vi "odczyt listy zdjec.vi"(5 "error in (no error)":errorcluster) -> (0 "error out":errorcluster, 1 "Nr zdjecia":i32[](array[numeric]), 2 "fps":i32[](array[numeric]), 3 "lista zdjec":string[](array[string]), 4 "sciezka do zdjec":path caption="selected path", 6 "godzina ze zdjecia":string[](array[string]))   [LabVIEW 2009]
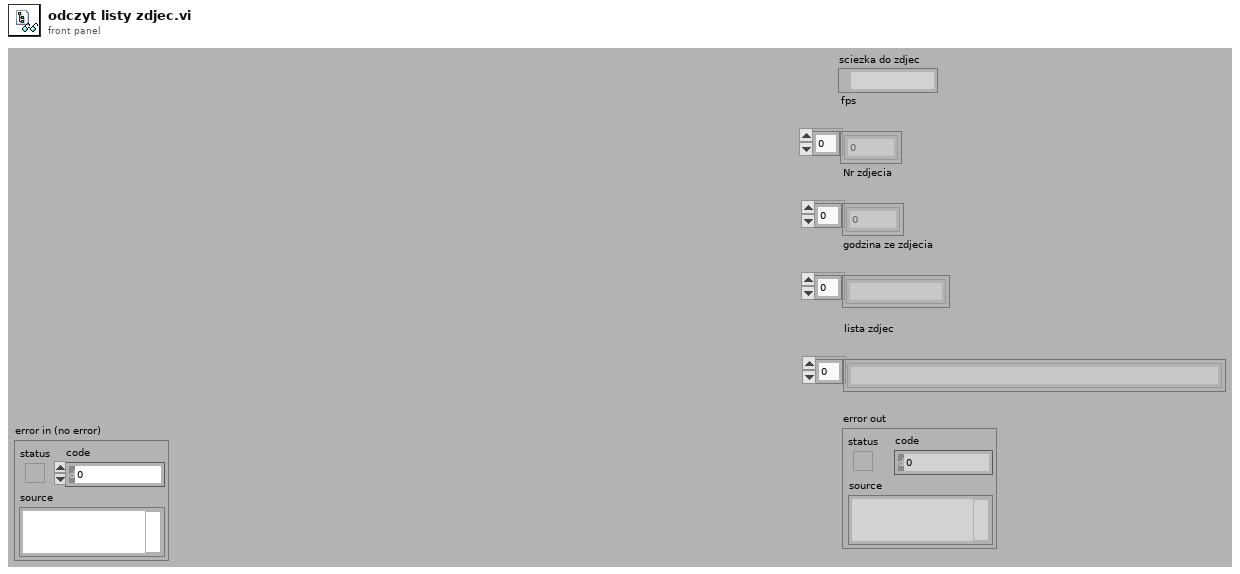
[diagram p1: front panel]
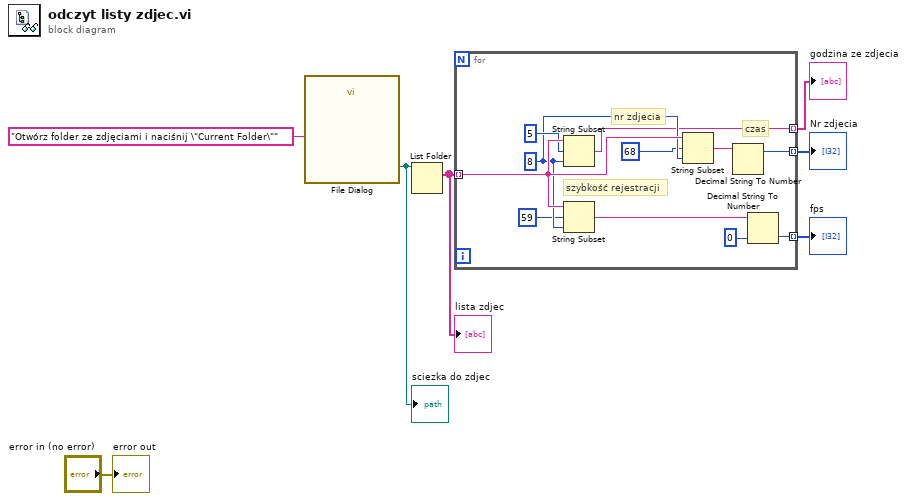
[diagram p0: block diagram]
diagram:
  n1 = call "File Dialog"("prompt"="Otwórz folder ze zdjęciami i naciśnij \"Current Folder\"") -> ("selected path"=w7:path)  [unwired: 11 in, 3 out]
  "sciezka do zdjec" <- w7
  n2 = List Folder(path=w7) -> (filenames=w5:string[])  [unwired: 3 in, 3 out]
  "lista zdjec" <- w5
  n3 = for {
    tunnel: w5 -> [w18] mode=indexing
    tunnel: [w8] -> w4 mode=indexing
    tunnel: [w10] -> w3 mode=indexing
    tunnel: [w11] -> w2 mode=indexing
    w16 = 8 ("length (rest)")
    # "nr zdjecia"
    # "szybkość rejestracji"
    # "czas"
    n4 = String Subset(string=w18, offset (0)=5, length (rest)=w16) -> (substring=w11:string)
    n5 = String Subset(string=w18, offset (0)=59, length (rest)=w16) -> (substring=w12:string)
    n6 = String Subset(string=w18, offset (0)=68, length (rest)=w16) -> (substring=w13:string)
    n7 = Decimal String To Number(string=w13) -> (offset past number=w8:i32)  [unwired: 2 in, 1 out]
    n8 = Decimal String To Number(string=w12, default (0L)=0 ("default (0 DBL)")) -> (number=w10:i32)  [unwired: 1 in, 1 out]
  }
  "godzina ze zdjecia" <- w2
  "fps" <- w3
  "Nr zdjecia" <- w4
  "error out" <- "error in (no error)"
